vi "qTVI.vi"(0 "System no.":i32=1 min=1 max=4 step=1, 3 "Invert order":bool, 5 "error in":errorcluster) -> (14 "Valid axis IDs":string[](array[string]), 19 "error out":errorcluster)   [LabVIEW 2020]
doc: "GCS 1.0: Get valid axis identifiers. Should be called before axes are renamed with SAI.vi. \nGCS 2.0: Get valid characters for axis IDs.\n\nC-702, C-848, C-880: Invert order should be TRUE. Returns valid axis identifiers. \n\nC-843, C-843.PM, C-844, C-865, C-866, E-710, E-761, Mercury: Invert order must be FALSE. Returns valid axis identifiers. \n\nC-867, C-877, C-884, C-891, E-135, E-517, E-518, E-871, E-872, E-873, E-874, Hydra, Pollux, Mercury_GCS: Invert order must be FALSE. Returns valid characters for axis IDs."
panel:
  # "GCS 1.0: Get valid axis identifiers. Should be called before\naxes are renamed with SAI.vi. \nGCS 2.0: Get valid characters for axis IDs.\nEXCEPTION: With this driver set, the ASCII characters\n{[}, {]} and {$} are not valid axis IDs."
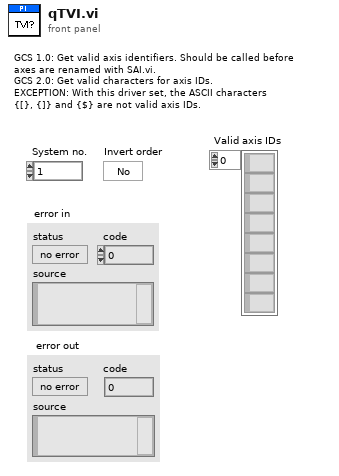
[diagram p1: front panel]
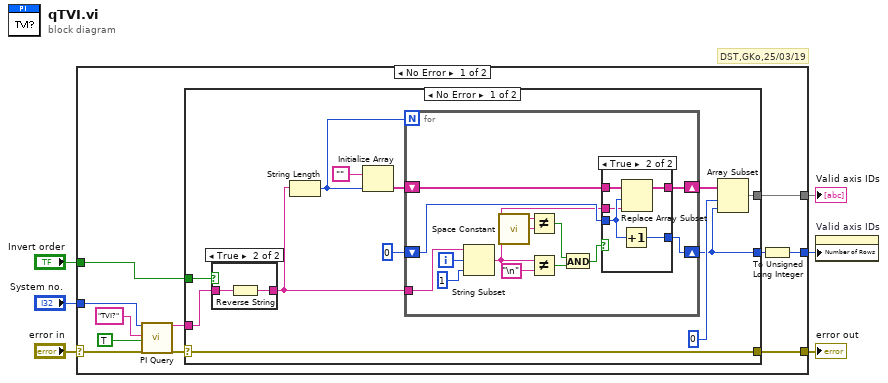
[diagram p0: block diagram]
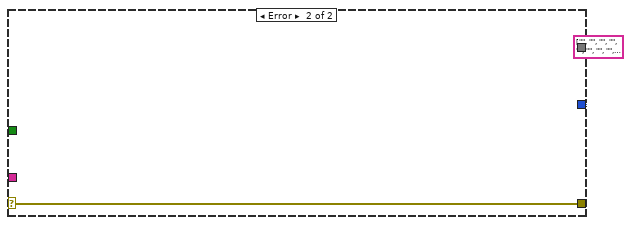
[diagram p4: hidden frame]
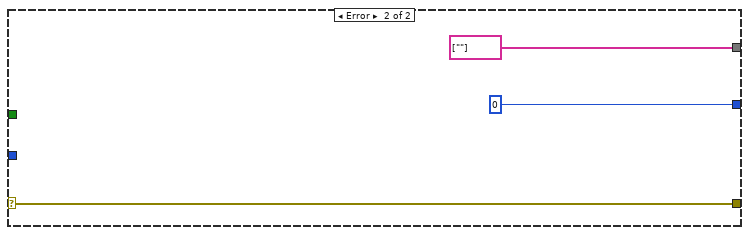
[diagram p5: hidden frame]
diagram:
  # "DST,GKo,25/03/19"
  n1 = case shown="No Error" "error in" {
    selector: "error in" -> [w12 w58]
    tunnel: "Invert order" -> [w7 _]
    tunnel: [w8 u32 0] -> w5
    tunnel: "System no." -> [w14 _]
    tunnel: [w13 string[] [""] ("Conn. Axes 2")] -> w3
    tunnel: [w9 w58] -> w2
    frame No Error {
      n2 = call "PI Query.vi"("System no."=w14, "String to send"="TVI?", "Attach termination char.?"=TRUE ("Attach Linefeed?"), "error in"=w12) -> ("String read"=w11:string, "error out"=w10:errorcluster)  [unwired: 3 in, 11 out]
      n3 = case shown="No Error" w10 {
        selector: w10 -> [w19 w53]
        tunnel: [w24 0] -> w15
        tunnel: [w22 string[] ["", "", "", "", "", "", "", "", "", "", "", "", "", "", "", "", "", "", "", "", "", "", "", "", "", "", ""] ("Conn. Axes 2")] -> w13
        tunnel: w11 -> [w20 _]
        tunnel: [w19 w53] -> w9
        tunnel: w7 -> [w18 _]
        frame No Error {
          n4 = case shown="True" w18 {
            tunnel: w20 -> [w30 w32]
            tunnel: [w30 w31] -> w21
            frame False {
            }
            frame True {
              n5 = Reverse String(1:w32) -> (0:w31:string)
            }
          }
          n6 = String Length(string=w21) -> (length=w28:i32)
          n7 = Initialize Array("" ("Element Data"), w28) -> (w26:string[])
          n8 = for {
            N: w28 -> [_]
            tunnel: w21 -> [w45]
            shift-right: [w38] -> w23
            shift-left: w26 -> [w39]
            shift-right: [w41] -> w24
            shift-left: 0 -> [w40]
            i -> [w43]
            n9 = String Subset(string=w45, offset (0)=w43, length (rest)=1 ("length")) -> (substring=w37:string)
            n10 = call <vilib>:"Space Constant.vi"() -> ("String"=w42:string)
            n11 = Not Equal?(x=w37, y=w42) -> (x != y?=w35:bool)
            n12 = Not Equal?(x=w37, y="\n") -> (x != y?=w34:bool)
            n13 = And(x=w35, y=w34) -> (x .and. y?=w33:bool)
            n14 = case shown="True" w33 {
              tunnel: [w47 w52] -> w41
              tunnel: w40 -> [w47 w50]
              tunnel: w39 -> [w46 w51]
              tunnel: w37 -> [_ w49]
              tunnel: [w46 w48] -> w38
              frame False {
              }
              frame True {
                n15 = Increment(x=w50) -> (x+1=w52:i32)
                n16 = Replace Array Subset(array=w51, new element=w49, index=w50) -> (w48:string[])
              }
            }
          }
          n17 = Array Subset(array=w23, index=0 ("Array Index"), length=w24) -> (w22:string[])
        }
        frame Error {
        }
      }
      n18 = To Unsigned Long Integer(number=w15) -> (unsigned 32bit integer=w8:u32)
    }
    frame Error {
    }
  }
  "error out" <- w2
  "Valid axis IDs" <- w3
  n19 = property on="Valid axis IDs" class="Arr (strict)"("Number of Rows"=w5) -> ()  [unwired: 2 in, 2 out]
